vi "Instrumentation LabJack Stream.vi"() -> ()   [LabVIEW 2020]
uses:
  <vilib>/Waveform/WDTOps.llb/WDT Get Waveform Time Array DBL.vi
panel:
  out "Stream Parameters":T1 {"Device Backlog [%]" format="%.2f"}
  out "Oxidizer Mass Flow":dynamicdata(graph)
  out "Pressure Chart":dynamicdata(graph)
  out "N2O Tank Mass":dynamicdata(graph)
  out "Tank Pressure":dbl(knob) scale=0.0..900.0
  out "Combustion Chamber Pressure":dbl(knob) scale=0.0..900.0
  out "N2O Tank Mass":dbl(slide) scale=17.0..21.0
  out "Grain Center":dbl(slide) scale=-70.0..40.0
  out "Post-Combustion":dbl(slide) scale=-70.0..40.0
  out "Pre-Combustion":dbl(slide) scale=-70.0..40.0
  out "Tank":dbl(slide) scale=-70.0..40.0
  in  "AIN Range":u8(ring) items=["LJ_rgBIP10V", "LJ_rgBIP1V", "LJ_rgBIPP1V", "LJ_rgBIPP01V"]
  in  "Display Rate (Hz)":i32=1
  in  "Binary":bool
  in  "StreamSettlingFactor":i32
  in  "Resolution Index":u8
  in  "PC buffer size (seconds)":dbl=10.0 format="%.2f"
  in  "Scan Rate (Hz)":dbl=1000.0 format="%.3f"
  in  "STOP":bool
  in  "Get Voltage":bool
  in  "Injector":string
  in  "Orifice Size":string
  in  "File Path Control":path
  out "Boolean":bool
  in  "Record Button":bool
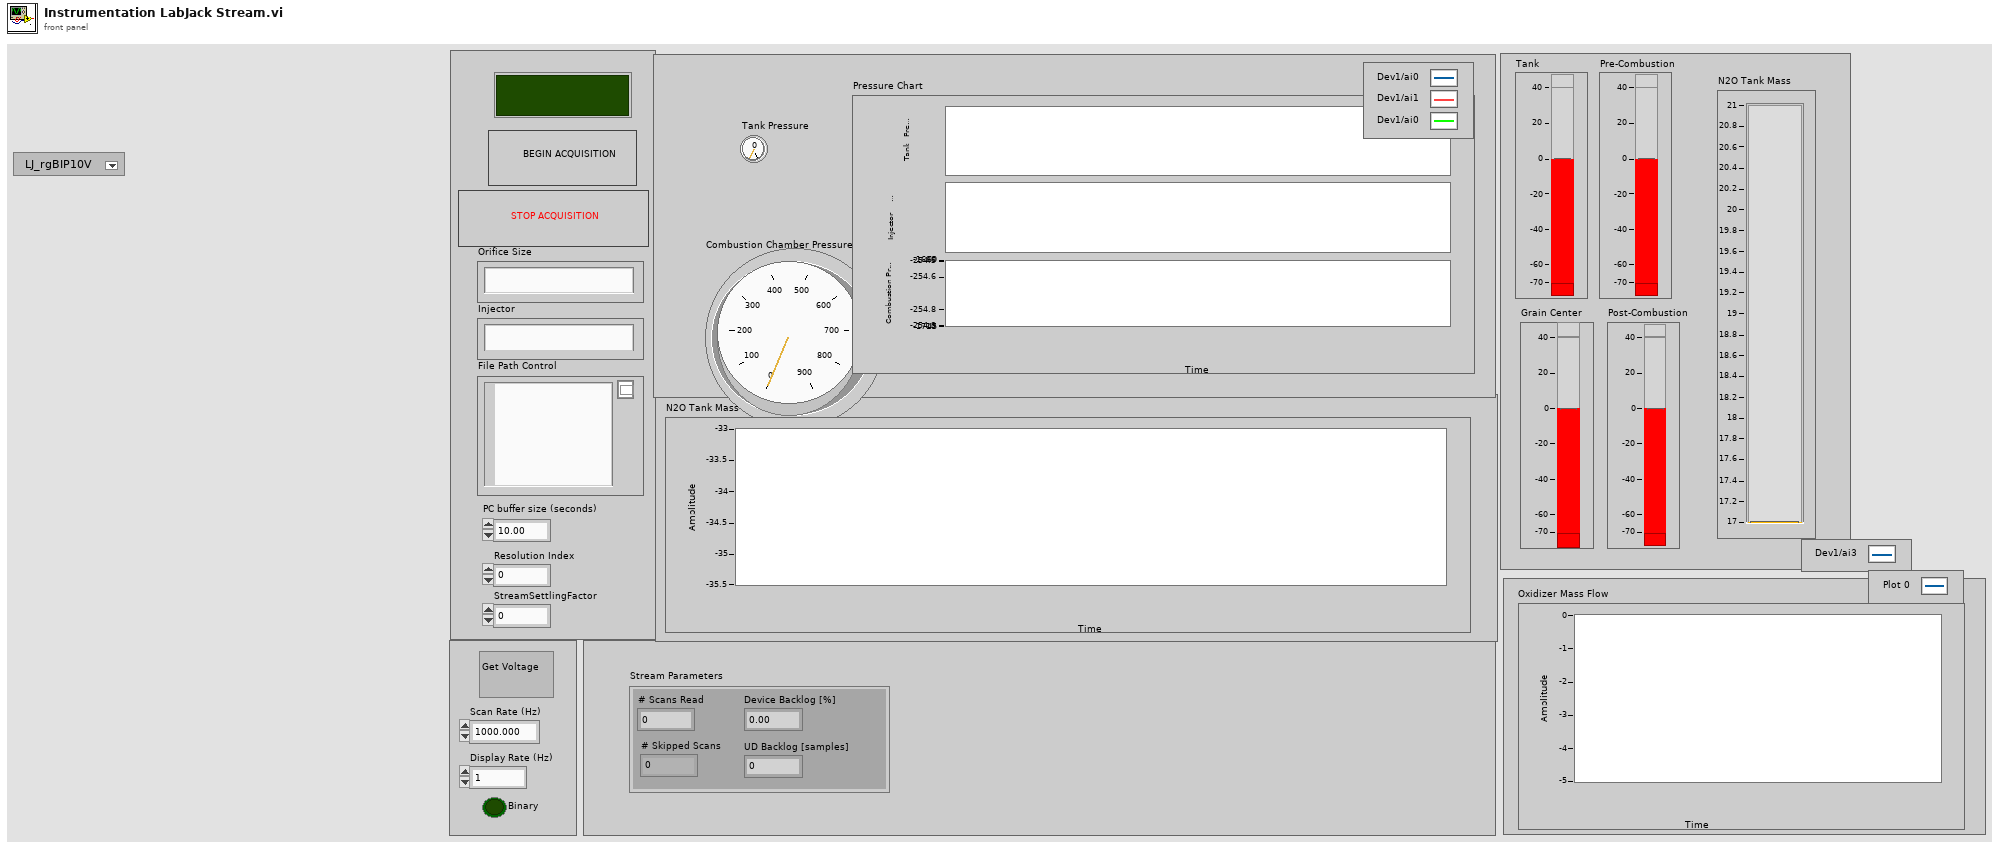
[diagram p1: front panel]
types:
  T1 = cluster{"# Scans Read":i32, "# Skipped Scans":i32, "Device Backlog [%]":dbl, "UD Backlog [samples]":i32}
  T2 = enum16{"open", "open or create", "create or replace", "create", "open (read-only)"}
  T3 = cluster{"PC buffer size (seconds)":dbl, "Resolution Index":u8, "StreamSettlingFactor":i32, "Binary":bool}
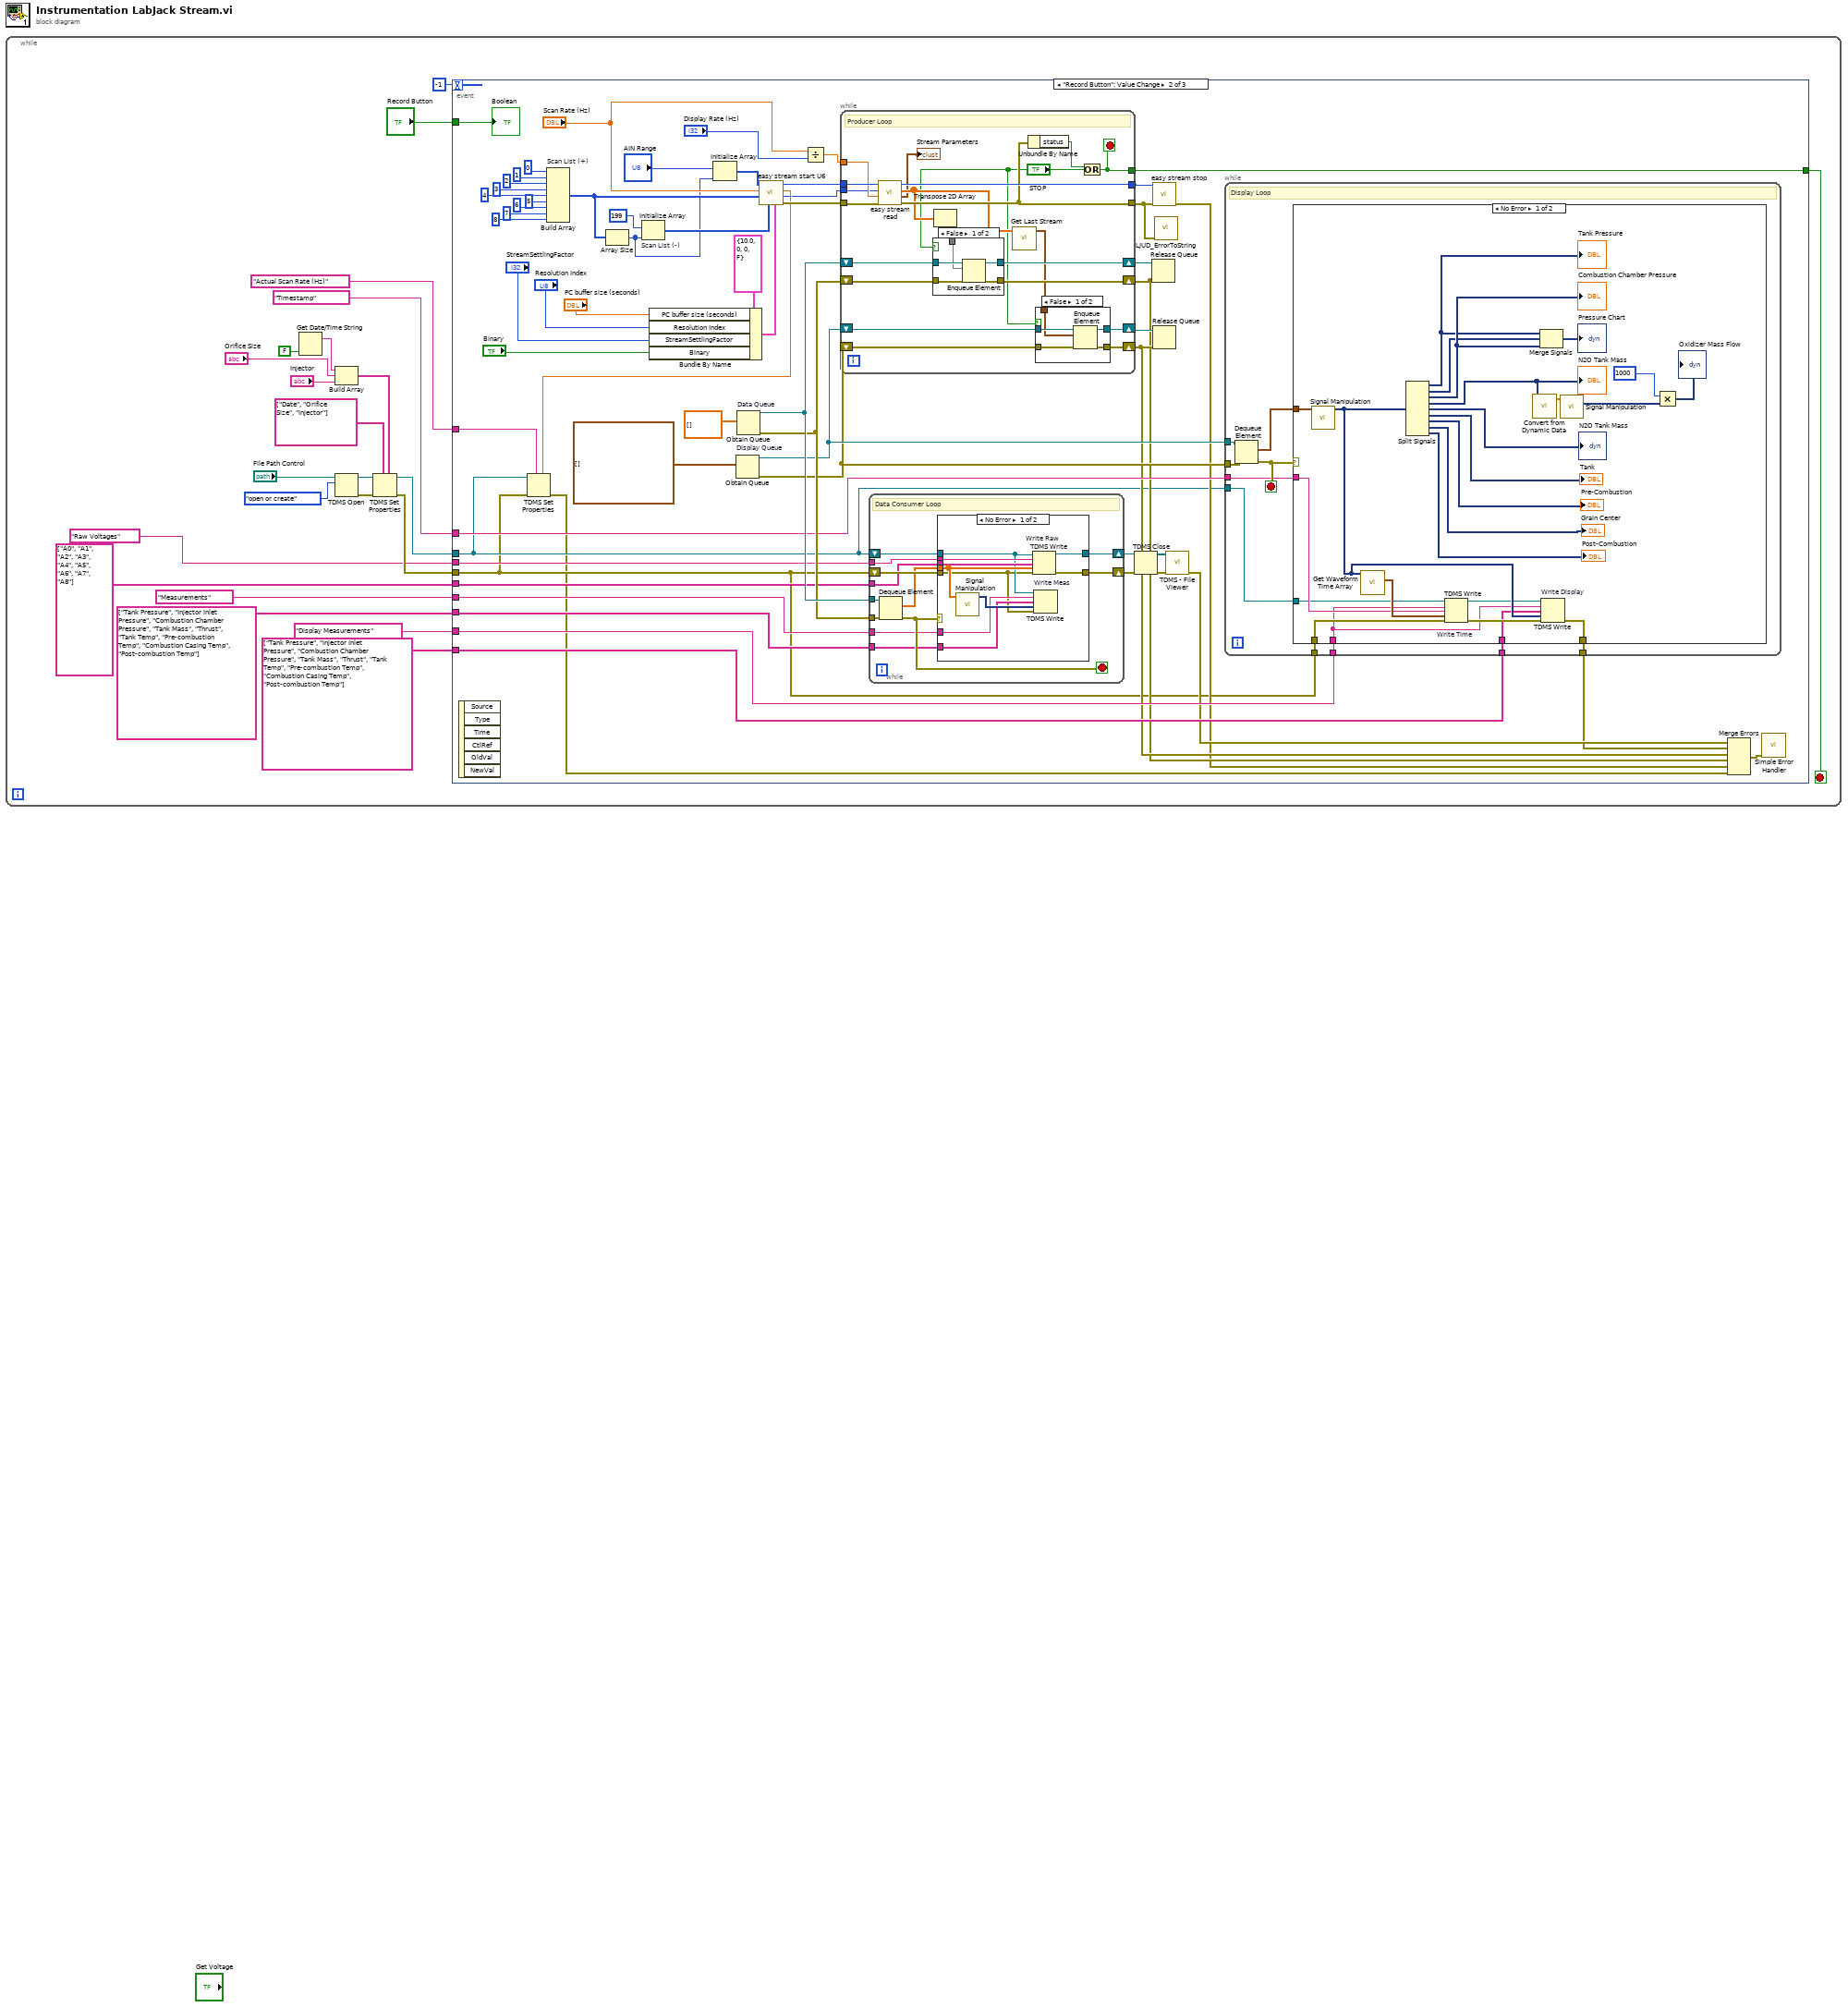
[diagram p0: block diagram]
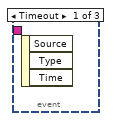
[diagram p2: hidden frame]
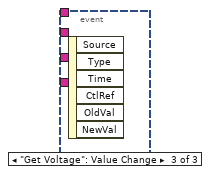
[diagram p7: hidden frame]
diagram:
  n1 = while {
    stop <- w9 stop-if-true
    n2 = Get Date/Time String(want seconds? (F)=FALSE) -> (date string=w19:string)  [unwired: 2 in, 1 out]
    n3 = Build Array(w19, "Orifice Size", "Injector") -> (w17:string[])
    n4 = TDMS Open(10:T2."open or create" ("operation (0:open)"), 11:"File Path Control") -> (0:w23:errorcluster, 3:w22:refnum<k34>)  [unwired: 5 in]
    n5 = TDMS Set Properties(5:w17, 7:string[] ["Date", "Orifice Size", "Injector"] ("property names"), 8:w23, 11:w22) -> (0:w12:errorcluster, 3:w10:refnum<k34>)  [unwired: 2 in, 2 out]
    n6 = event shown="[1] \"Record Button\": Value Change" {
      selector: _ -> [_ _ _]
      dyn-events: _ -> [_ _ _]
      timeout: -1 -> [_ _ _]
      tunnel: w12 -> [_ w29 _]
      tunnel: "Record Button" -> [_ w44 _]
      tunnel: w10 -> [_ w30 _]
      tunnel: [_ w45 _] -> w9
      tunnel: "Raw Voltages" -> [_ w43 _]
      tunnel: string[] ["A0", "A1", "A2", "A3", "A4", "A5", "A6", "A7", "A8"] ("property names") -> [_ w42 _]
      tunnel: "Measurements" -> [_ w41 _]
      tunnel: string[] ["Tank Pressure", "Injector Inlet Pressure", "Combustion Chamber Pressure", "Tank Mass", "Thrust", "Tank Temp", "Pre-combustion Temp", "Combustion Casing Temp", "Post-combustion Temp"] ("property names") -> [_ w40 _]
      tunnel: "Display Measurements" -> [_ w39 _]
      tunnel: "Timestamp" -> [_ w38 _]
      tunnel: string[] ["Tank Pressure", "Injector Inlet Pressure", "Combustion Chamber Pressure", "Tank Mass", "Thrust", "Tank Temp", "Pre-combustion Temp", "Combustion Casing Temp", "Post-combustion Temp"] ("property names") -> [_ w37 _]
      tunnel: "Actual Scan Rate (Hz)" -> [_ w27 _]
      event Timeout {
        n7 = event-data() -> ()  [unwired: 1 in, 3 out]
      }
      event "Record Button": Value Change {
        n8 = event-data() -> ()  [unwired: 1 in, 6 out]
        n9 = Build Array "Scan List (+)"(0 ("SettlingFactor"), 1 ("SettlingFactor"), 2 ("SettlingFactor"), 3 ("SettlingFactor"), 4 ("SettlingFactor"), 5 ("SettlingFactor"), 6 ("SettlingFactor"), 7 ("SettlingFactor"), 8 ("SettlingFactor")) -> (w57:i32[])
        n10 = Array Size(array=w57) -> (size(s)=w55:i32)
        n11 = Initialize Array "Scan List (-)"(199, w55) -> (w59:i32[])
        n12 = Bundle By Name(cluster=T3 {"PC buffer size (seconds)"=10.0, "Resolution Index"=0, "StreamSettlingFactor"=0, "Binary"=FALSE} ("Advanced"), "PC buffer size (seconds)"="PC buffer size (seconds)", "Resolution Index"="Resolution Index", "StreamSettlingFactor"="StreamSettlingFactor", "Binary"="Binary") -> (w74:T3)
        n13 = Initialize Array("AIN Range", w55) -> (w56:u8[])
        n14 = Obtain Queue "Display Queue"(element data type=waveform(dbl)[] []) -> (queue out=w47:refnum<queue>, error out=w46:errorcluster)  [unwired: 4 in, 1 out]
        n15 = Obtain Queue "Data Queue"(element data type=dbl[][] []) -> (queue out=w52:refnum<queue>, error out=w51:errorcluster)  [unwired: 4 in, 1 out]
        n16 = call "easy stream start U6.vi"("Advanced"=w74, "Scan List (-)"=w59, "Scan List (+)"=w57, "Scan Rate (Hz)"="Scan Rate (Hz)", "Range Constants"=w56) -> ("error out"=w70:errorcluster, "# Channels"=w24:i32, "Actual Scan Rate (Hz)"=w26:dbl, "Handle Out"=w72:i32)  [unwired: 3 in]
        n17 = TDMS Set Properties(5:w26, 7:w27, 8:w29, 11:w30) -> (0:w28:errorcluster)  [unwired: 2 in, 3 out]
        n18 = Divide(x="Scan Rate (Hz)", y="Display Rate (Hz)") -> (x/y=w71:dbl)
        n19 = while {
          tunnel: w72 -> [w165]
          tunnel: w71 -> [w164]
          tunnel: w24 -> [w163]
          tunnel: [w161] -> w69
          tunnel: [w158] -> w45
          tunnel: w70 -> [w162]
          tunnel: [w160] -> w68
          shift-right: [w157] -> w53
          shift-left: w52 -> [w156]
          shift-right: [w154] -> w32
          shift-left: w51 -> [w155]
          shift-right: [w148] -> w48
          shift-left: w47 -> [w151]
          shift-right: [w147] -> w33
          shift-left: w46 -> [w149]
          stop <- w158 stop-if-true
          # "Producer Loop"
          n20 = call "easy stream read.vi"("error in"=w162, "Scans To Read"=w164, "# Channels In Stream"=w163, "Handle In"=w165) -> ("error out"=w160:errorcluster, "Stream Parameters"=→"Stream Parameters":T1, "Data"=w152:dbl[][], "Handle Out"=w161:i32)  [unwired: 4 in]
          n21 = Transpose 2D Array(2D array=w152) -> (transposed array=w153:dbl[][])
          n22 = case shown="False" "STOP" {
            tunnel: [w175 w179] -> w157
            tunnel: w156 -> [w177 w179]
            tunnel: w155 -> [w176 w178]
            tunnel: w153 -> [w174 _]
            tunnel: [w173 w178] -> w154
            frame False {
              n23 = Enqueue Element(queue=w177, element=w174, error in (no error)=w176) -> (queue out=w175:refnum<queue>, error out=w173:errorcluster)  [unwired: 1 in, 1 out]
            }
            frame True {
            }
          }
          n24 = call "Get Last Stream.vi"("Data"=w152) -> ("Array of Waveform"=w150:waveform(dbl)[])  [unwired: 10 in]
          n25 = Unbundle By Name(w160) -> ("status"=w159:bool)
          n26 = case shown="False" "STOP" {
            tunnel: w151 -> [w170 w172]
            tunnel: w150 -> [w169 _]
            tunnel: w149 -> [w168 w171]
            tunnel: [w167 w172] -> w148
            tunnel: [w166 w171] -> w147
            frame False {
              n27 = Enqueue Element(queue=w170, element=w169, error in (no error)=w168) -> (queue out=w167:refnum<queue>, error out=w166:errorcluster)  [unwired: 1 in, 1 out]
            }
            frame True {
            }
          }
          n28 = Or(x=w159, y="STOP") -> (x .or. y?=w158:bool)
        }
        n29 = while {
          tunnel: w43 -> [w131]
          tunnel: w42 -> [w130]
          shift-right: [w123] -> w82
          shift-left: w29 -> [w132]
          shift-right: [w124] -> w81
          shift-left: w30 -> [w129]
          tunnel: w52 -> [w128]
          tunnel: w51 -> [w127]
          tunnel: w41 -> [w122]
          tunnel: w40 -> [w121]
          stop <- w126 stop-if-true
          # "Data Consumer Loop"
          n30 = Dequeue Element(queue=w128, error in (no error)=w127) -> (element=w125:dbl[][], error out=w126:errorcluster)  [unwired: 1 in, 2 out]
          n31 = case shown="No Error" w126 {
            tunnel: w132 -> [w133 w143]
            tunnel: w131 -> [w142 _]
            tunnel: w130 -> [w141 _]
            tunnel: w129 -> [w136 w144]
            tunnel: w125 -> [w138 _]
            tunnel: [w140 w144] -> w124
            tunnel: [w139 w143] -> w123
            tunnel: w122 -> [w135 _]
            tunnel: w121 -> [w134 _]
            frame No Error {
              n32 = call "Signal Manipulation.vi"("Tank Mass"=w138) -> ("Dynamic Data"=w137:dynamicdata)  [unwired: 10 in]
              n33 = TDMS Write "Write Raw"(0:w136, 5:w142, 7:w141, 9:w138, 11:w133) -> (4:w140:refnum<k34>, 15:w139:errorcluster)  [unwired: 1 in, 2 out]
              n34 = TDMS Write "Write Meas"(0:w136, 5:w135, 7:w134, 9:w137, 11:w133) -> ()  [unwired: 1 in, 4 out]
            }
            frame Error {
            }
          }
        }
        n35 = TDMS Close(8:w82, 11:w81) -> (0:w84:errorcluster, 3:w83:path)
        n36 = Release Queue(queue=w53, error in (no error)=w32) -> ()  [unwired: 1 in, 3 out]
        n37 = call "easy stream stop.vi"("error in"=w68, "Handle In"=w69) -> ("error out"=w31:errorcluster)  [unwired: 7 in, 2 out]
        n38 = Release Queue(queue=w48, error in (no error)=w33) -> ()  [unwired: 1 in, 3 out]
        n39 = call "LJUD_ErrorToString.vi"("error in"=w68) -> ()  [unwired: 10 in, 1 out]
        n40 = call <vilib>:"TDMS - File Viewer.vi"("error in (no error)"=w84, "file path"=w83) -> ("error out"=w35:errorcluster)  [unwired: 4 in, 1 out]
        n41 = while {
          tunnel: w47 -> [w92]
          tunnel: w46 -> [w91]
          tunnel: w39 -> [w90]
          tunnel: w38 -> [w89]
          tunnel: w29 -> [w88]
          tunnel: w30 -> [w87]
          tunnel: w37 -> [w86]
          tunnel: [w85] -> w34
          stop <- w94 stop-if-true
          # "Display Loop"
          n42 = Dequeue Element(queue=w92, error in (no error)=w91) -> (element=w93:waveform(dbl)[], error out=w94:errorcluster)  [unwired: 1 in, 2 out]
          n43 = case shown="No Error" w94 {
            tunnel: w93 -> [w97 _]
            tunnel: w90 -> [w102 _]
            tunnel: w89 -> [w107 _]
            tunnel: w88 -> [w106 w120]
            tunnel: w87 -> [w104 _]
            tunnel: w86 -> [w101 _]
            tunnel: [w100 w120] -> w85
            frame No Error {
              n44 = call "Signal Manipulation.vi"("Tank Mass"=w97) -> ("Dynamic Data"=w109:dynamicdata)  [unwired: 10 in]
              n45 = call-poly <vilib>:"Get Waveform Time Array.vi"("waveform in"=w109) -> ("X array"=w108:timestamp[])  [unwired: 9 in, 1 out]
              n46 = Split Signals(w109) -> (w99:dynamicdata, w98:dynamicdata, w115:dynamicdata, w114:dynamicdata, →"N2O Tank Mass":dynamicdata, →"Tank":dynamicdata, →"Pre-Combustion":dynamicdata, →"Grain Center":dynamicdata, →"Post-Combustion":dynamicdata)  [unwired: 9 in]
              "N2O Tank Mass" <- w114
              "Combustion Chamber Pressure" <- w115
              "Tank Pressure" <- w99
              n47 = TDMS Write "Write Time"(0:w104, 5:w102, 7:w107, 9:w108, 11:w106) -> (4:w103:refnum<k34>, 15:w105:errorcluster)  [unwired: 1 in, 2 out]
              n48 = call "Convert from Dynamic Data"("Dynamic Data Type"=w114) -> ("Array"=w95:dbl[])  [unwired: 3 in]
              n49 = Merge Signals(w99, w98, w115) -> (→"Pressure Chart":dynamicdata)
              n50 = TDMS Write "Write Display"(0:w103, 5:w102, 7:w101, 9:w109, 11:w105) -> (15:w100:errorcluster)  [unwired: 1 in, 3 out]
              n51 = call "Signal Manipulation.vi"("Tank Mass"=w95) -> ("Dynamic Data"=w116:dynamicdata)  [unwired: 10 in]
              n52 = Multiply(x=1000, y=w116) -> (x*y=→"Oxidizer Mass Flow":dynamicdata)
            }
            frame Error {
            }
          }
        }
        n53 = Merge Errors(w35, w34, w33, w32, w31, w28) -> (w36:errorcluster)
        n54 = call <vilib>:"Simple Error Handler.vi"("error in (no error)"=w36) -> ()  [unwired: 2 in, 7 out]
        "Boolean" <- w44
      }
      event "Get Voltage": Value Change {
        n55 = event-data() -> ()  [unwired: 1 in, 6 out]
      }
    }
  }
